vi "Periodic Tasks.vi"(8 "error in":errorcluster) -> ()   [LabVIEW 2013]
doc: "This VI runs in parallel to other tasks. It can contain as many user-defined periodic loops as you need. These can carry out PID or other sorts of timed response."
uses:
  <vilib>/Rock Robotics/WPI/Ultrasonic/WPI_UltrasonicRangeUnits.ctl
  <vilib>/Rock Robotics/SystemInterfaces/Utilities/FPGA_UtilitiesLED Source.ctl
  <vilib>/Rock Robotics/SystemInterfaces/Utilities/FPGA_UtilitiesLED State.ctl
  <vilib>/Rock Robotics/WPI/Relay/WPI_RelayValue.ctl
  <vilib>/Rock Robotics/WPI/DriverStation/WPI_DriverStationRobotMode2.ctl
  <vilib>/Rock Robotics/WPI/Solenoid/WPI_SolenoidValue.ctl
  <vilib>/Rock Robotics/WPI/Compressor/WPI_CompressorGetSetRefNum.vi
  Robot Global Data.vi
  <vilib>/Rock Robotics/WPI/Solenoid/WPI_SolenoidSetEnum.vi
panel:
  out "Shooter up":bool
  in  "Winch":bool
  in  "Bola coletada?":bool
  in  "Em posicao?":bool
  in  "upper limit":dbl=100.0
  in  "lower limit":dbl=60.0
  in  "milliseconds to wait":u32=1000
  out "Motor garra 2":dbl
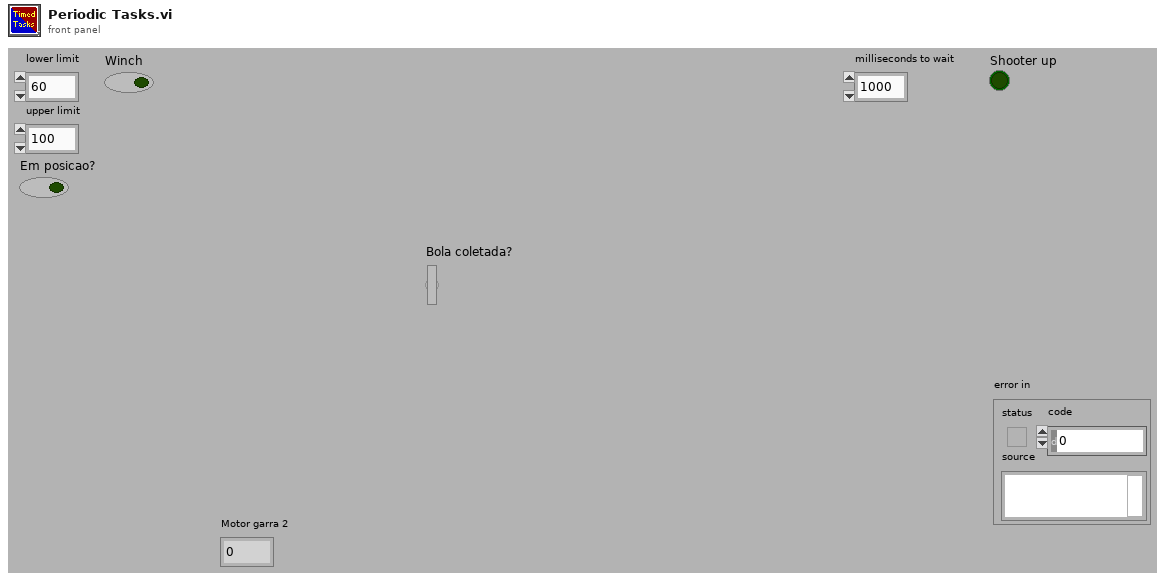
[diagram p1: front panel]
types:
  T1 = typedef "WPI_DriverStationRobotMode2.ctl" = enum16{"Autonomous Disabled", "Autonomous Enabled", "Teleop Disabled", "Teleop Enabled", "Timeout", "Finish", "Test Disabled", "Test Enabled"}
  T2 = typedef "WPI_DigitalInputDevRef.ctl" = cluster{"DevStatus":errorcluster, "DIO Channel":T3, "Digital Module":T4}
  T3 = typedef "FPGA_DIOChannel.ctl" = enum8{"DIO 1", "DIO 2", "DIO 3", "DIO 4", "DIO 5", "DIO 6", "DIO 7", "DIO 8", "DIO 9", "DIO 10", "DIO 11", "DIO 12", "DIO 13", "DIO 14", "Invalid"}
  T4 = typedef "FPGA_TypedefDigitalModule.ctl" = enum16{"Digital Module 1", "Digital Module 2"}
  T5 = typedef "WPI_MotorControlDeviceRef.ctl" = cluster{"DeviceStatus":errorcluster, "Type":enum16{"PWM", "CAN"}, "PWM":cluster{"Digital Module":T4, "PWM Channel":T6, "DeadBand":T7}, "CAN":cluster{"Device Number":u8, "Control Mode":T8, "Semaphore":T9, "Max Vout":dbl}, "Invert":bool, "TransformRef":T10, "InvTransformRef":T10}
  T6 = typedef "FPGA_DIOPWMChannel.ctl" = enum8{"PWM 1", "PWM 2", "PWM 3", "PWM 4", "PWM 5", "PWM 6", "PWM 7", "PWM 8", "PWM 9", "PWM 10", "Invalid"}
  T7 = typedef "WPI_PWMDeadband.ctl" = cluster{"Name":string, "maxPositivePwm":i32, "minPositivePwm":i32, "centerPwm":i32, "maxNegativePwm":i32, "minNegativePwm":i32, "angularRange":u16}
  T8 = typedef "WPI_CANJaguar_ControlMode.ctl" = enum8{"Percent VBus", "Current", "Speed", "Position", "Voltage"}
  T9 = typedef "Semaphore RefNum" = refnum<k1>
  T10 = typedef "WPI_PWMTransform_ConPane.ctl" = refnum<vi>
  T11 = typedef "WPI_JoystickDevRef.ctl" = cluster{"Device":T12}
  T12 = typedef "WPI_JoystickDeviceEnum.ctl" = enum16{"USB 1", "USB 2", "USB 3", "USB 4", "Kinect 1", "Kinect 2"}
  T13 = typedef "WPI_JoystickButtonState.ctl" = cluster{"Button 1":bool, "Button 2":bool, "Button 3":bool, "Button 4":bool, "Button 5":bool, "Button 6":bool, "Button 7":bool, "Button 8":bool, "Button 9":bool, "Button 10":bool, "Button 11":bool, "Button 12":bool}
  T14 = typedef "WPI_CompressorDevRef.ctl" = cluster{"DevStatus":errorcluster, "DigitalInputDevRef":T2, "RelayDevRef":T15}
  T15 = typedef "WPI_RelayDevRef.ctl" = cluster{"DevStatus":errorcluster, "Relay Channel":T16, "Digital Module":T4, "Relay Direction":T17}
  T16 = typedef "FPGA_DIORelayChannel.ctl" = enum8{"Relay 1", "Relay 2", "Relay 3", "Relay 4", "Relay 5", "Relay 6", "Relay 7", "Relay 8", "Invalid"}
  T17 = typedef "WPI_RelayDirection.ctl" = enum16{"Both directions", "Forward only", "Reverse only"}
  T18 = typedef "WPI_SolenoidValue.ctl" = enum16{"Off", "On", "Forward", "Reverse"}
  T19 = typedef "WPI_SolenoidDevRef.ctl" = cluster{"DevStatus":errorcluster, "Solenoid Module":T20, "Forward Solenoid Channel":T21, "Reverse Solenoid Channel":T21}
  T20 = typedef "FPGA_TypedefSolenoidModule.ctl" = enum16{"Solenoid Module 1", "Solenoid Module 2"}
  T21 = typedef "WPI_SolenoidChannel.ctl" = enum8{"Solenoid 1", "Solenoid 2", "Solenoid 3", "Solenoid 4", "Solenoid 5", "Solenoid 6", "Solenoid 7", "Solenoid 8", "Invalid"}
  T22 = typedef "WPI_RelayValue.ctl" = enum16{"Off", "On", "Forward", "Reverse"}
  T23 = typedef "FPGA_UtilitiesLED State.ctl" = enum16{"Off", "On", "Toggle"}
  T24 = typedef "FPGA_UtilitiesLED Source.ctl" = enum16{"User LED", "FPGA LED"}
  T25 = typedef "WPI_UltrasonicDeviceRef.ctl" = cluster{"DevStatus":errorcluster, "Ping Digital Module":T4, "Echo Digital Module":T4, "Ping Channel":T3, "Echo Channel":T3, "CntIndex":T26}
  T26 = typedef "FPGA_CounterCtrSystemIndex.ctl" = enum8{"Ctr 0", "Ctr 1", "Ctr 2", "Ctr 3", "Ctr 4", "Ctr 5", "Ctr 6", "Ctr 7", "Invalid"}
  T27 = typedef "WPI_UltrasonicRangeUnits.ctl" = enum16{"inches", "mm"}
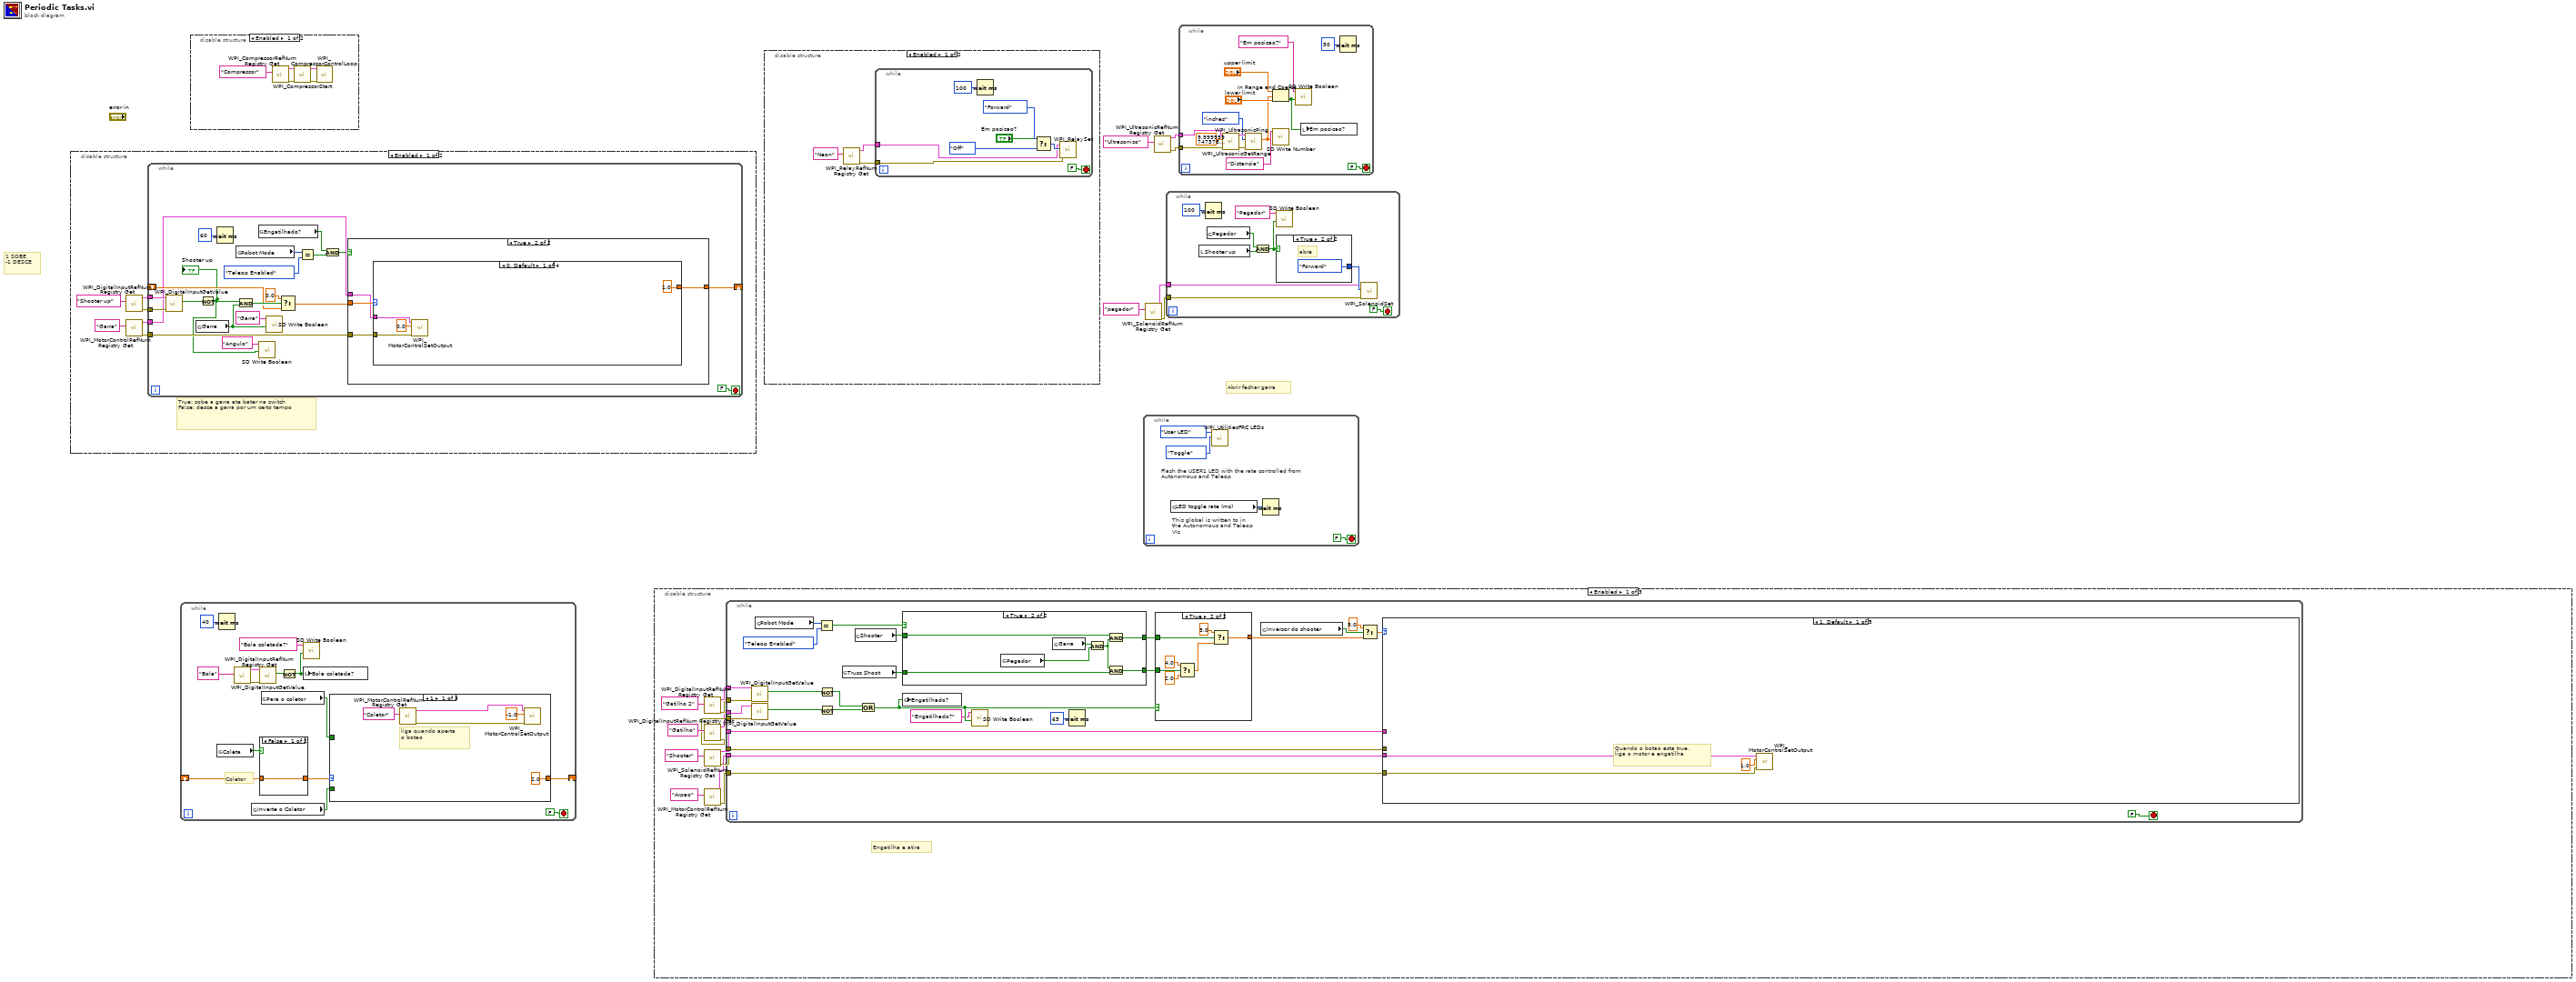
[diagram p0: block diagram]
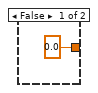
[diagram p4: hidden frame]
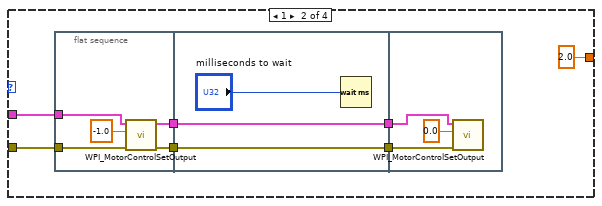
[diagram p5: hidden frame]
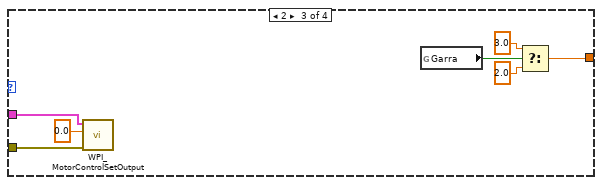
[diagram p6: hidden frame]
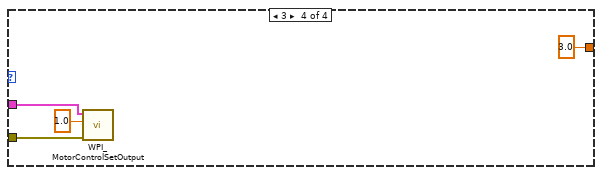
[diagram p7: hidden frame]
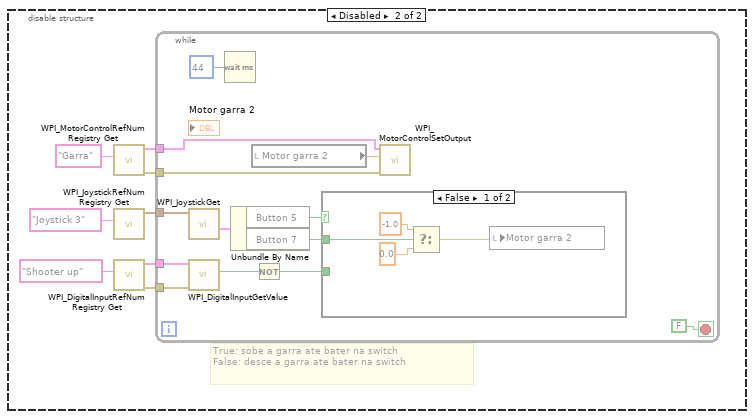
[diagram p8: hidden frame]
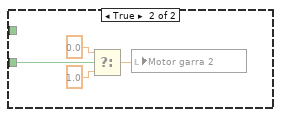
[diagram p9: hidden frame]
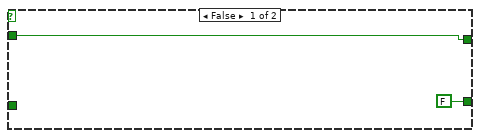
[diagram p10: hidden frame]
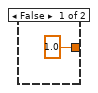
[diagram p11: hidden frame]
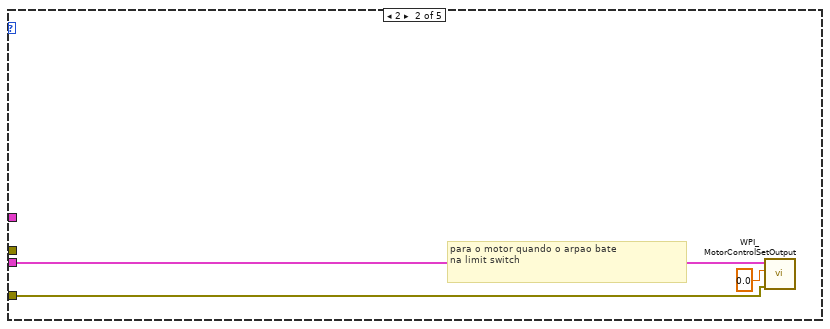
[diagram p12: hidden frame]
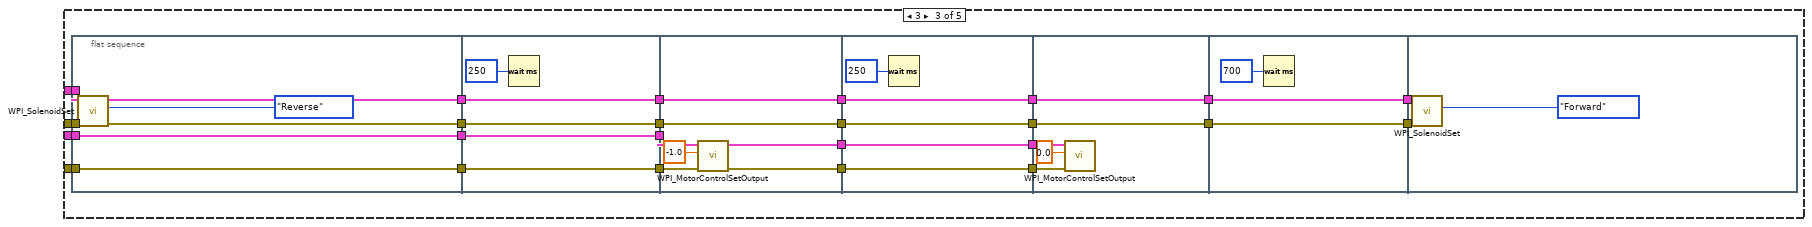
[diagram p13: hidden frame]
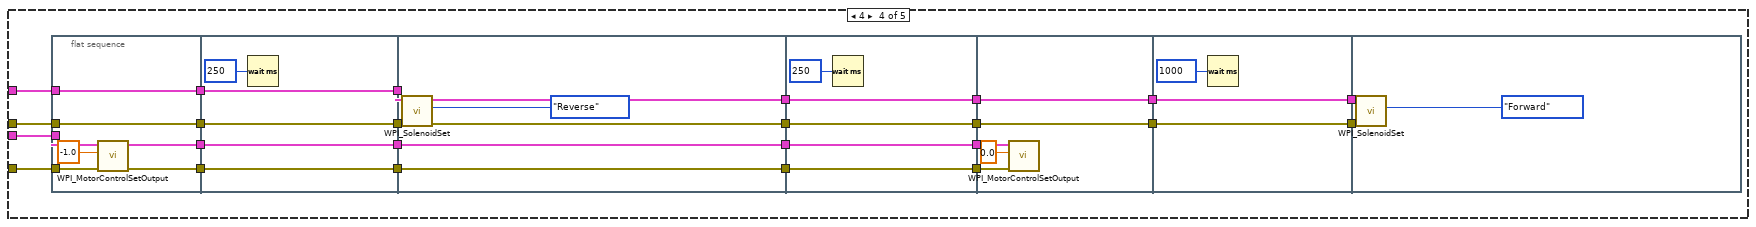
[diagram p14: hidden frame]
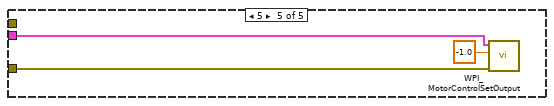
[diagram p15: hidden frame]
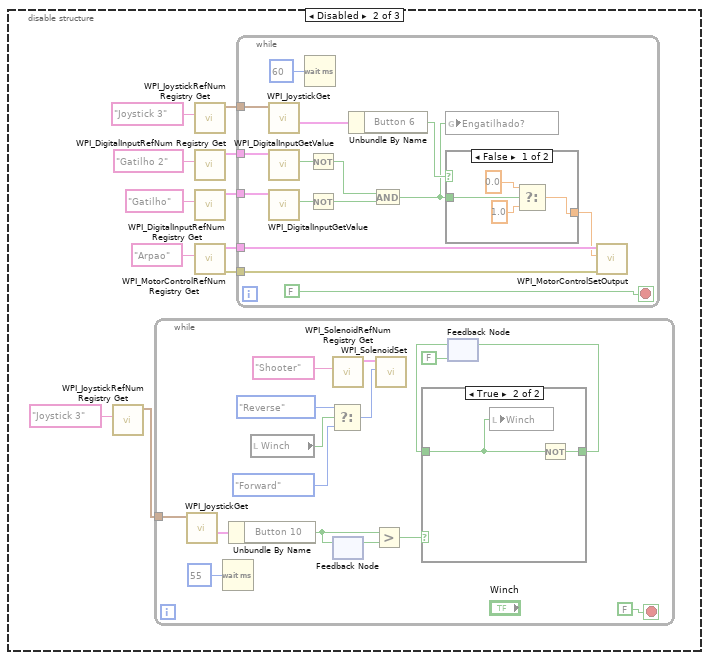
[diagram p16: hidden frame]
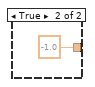
[diagram p18: hidden frame]
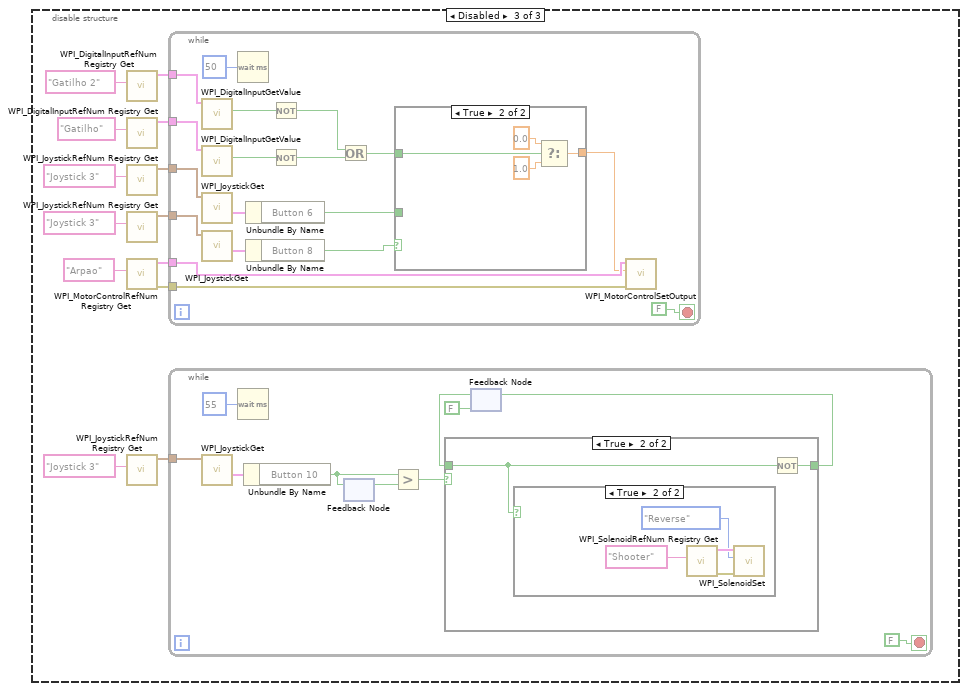
[diagram p19: hidden frame]
diagram:
  # "1 SOBE\n-1 DESCE"
  # "Abrir fechar garra"
  n1 = disable-structure shown="Enabled" {
    frame Enabled {
      # "True: sobe a garra ate bater na switch\nFalse: desce a garra por um certo tempo"
      n2 = call <vilib>:"WPI_DigitalInputRefNum Registry Get.vi"("refnum name"="Shooter up") -> ("error out"=w9:errorcluster, "DigitalInputDevRef"=w10:T2)  [unwired: 9 in]
      n3 = call <vilib>:"WPI_MotorControlRefNum Registry Get.vi"("refnum name"="Garra") -> ("error out"=w11:errorcluster, "MotorControlDevRef"=w12:T5)  [unwired: 9 in]
      n4 = while {
        tunnel: w12 -> [w24]
        tunnel: w11 -> [w23]
        tunnel: w10 -> [w32]
        tunnel: w9 -> [w31]
        shift-right: [w25] -> _
        shift-left: _ -> [w26]
        stop <- FALSE stop-if-true
        n5 = call <vilib>:"WPI_DigitalInputGetValue.vi"("error in (no error)"=w31, "DigitalInputDevRef"=w32) -> ("Value"=w22:bool)  [unwired: 7 in, 2 out]
        n6 = global read "Robot Global Data.vi" "Garra"() -> (w15:bool)
        n7 = Not(x=w22) -> (.not. x?=w13:bool)
        "Shooter up" <- w13
        n8 = Wait (ms)(milliseconds to wait=u32 60) -> ()  [unwired: 1 out]
        n9 = global read "Robot Global Data.vi" "Robot Mode"() -> (w20:T1)
        n10 = And(x=w13, y=w15) -> (x .and. y?=w29:bool)
        n11 = global read "Robot Global Data.vi" "Engatilhado?"() -> (w17:bool)
        n12 = call <vilib>:"SD Write Boolean.vi"("Boolean"=w13, "Name"="Angulo") -> ()  [unwired: 8 in, 2 out]
        n13 = call <vilib>:"SD Write Boolean.vi"("Boolean"=w15, "Name"="Garra") -> ()  [unwired: 8 in, 2 out]
        n14 = Select(t=0.0, s=w29, f=w26) -> (s? t:f=w27:dbl)
        n15 = Equal?(x=w20, y=WPI_DriverStationRobotMode2."Teleop Enabled") -> (x = y?=w18:bool)
        n16 = And(x=w17, y=w18) -> (x .and. y?=w16:bool)
        n17 = case shown="True" w16 {
          tunnel: w27 -> [_ w38]
          tunnel: [0.0 ("f") w37] -> w25
          tunnel: w24 -> [_ w36]
          tunnel: w23 -> [_ w35]
          frame False {
          }
          frame True {
            n18 = case shown="0, Default" w38 {
              tunnel: [1.0 ("Motor garra") 2.0 ("Motor garra") w65 3.0 ("f")] -> w37
              tunnel: w36 -> [w41 w48 w64 w69]
              tunnel: w35 -> [w40 w47 w63 w68]
              frame 0, Default {
                n19 = call <vilib>:"WPI_MotorControlSetOutput.vi"("error in (no error)"=w40, "Output"=0.0 ("Motor garra"), "MotorControlDevRef"=w41) -> ()  [unwired: 6 in, 3 out]
              }
              frame 1 {
                n20 = flat-sequence {
                  tunnel: w48 -> [w54]
                  tunnel: w47 -> [w53]
                  tunnel: [w51] -> w46
                  tunnel: [w50] -> w45
                  tunnel: [w57] -> w44
                  tunnel: w46 -> [w57]
                  tunnel: [w56] -> w43
                  tunnel: w45 -> [w56]
                  tunnel: w44 -> [w58]
                  tunnel: w43 -> [w60]
                  frame #0 {
                    n21 = call <vilib>:"WPI_MotorControlSetOutput.vi"("error in (no error)"=w53, "Output"=-1.0, "MotorControlDevRef"=w54) -> ("error out"=w50:errorcluster, "MotorControlDevRef"=w51:T5)  [unwired: 6 in, 1 out]
                  }
                  frame #1 {
                    n22 = Wait (ms)(milliseconds to wait="milliseconds to wait") -> ()  [unwired: 1 out]
                  }
                  frame #2 {
                    n23 = call <vilib>:"WPI_MotorControlSetOutput.vi"("error in (no error)"=w60, "Output"=0.0 ("f"), "MotorControlDevRef"=w58) -> ()  [unwired: 6 in, 3 out]
                  }
                }
              }
              frame 2 {
                n24 = call <vilib>:"WPI_MotorControlSetOutput.vi"("error in (no error)"=w63, "Output"=0.0 ("Motor garra"), "MotorControlDevRef"=w64) -> ()  [unwired: 6 in, 3 out]
                n25 = global read "Robot Global Data.vi" "Garra"() -> (w61:bool)
                n26 = Select(t=3.0, s=w61, f=2.0) -> (s? t:f=w65:dbl)
              }
              frame 3 {
                n27 = call <vilib>:"WPI_MotorControlSetOutput.vi"("error in (no error)"=w68, "Output"=1.0 ("Motor garra"), "MotorControlDevRef"=w69) -> ()  [unwired: 6 in, 3 out]
              }
            }
          }
        }
      }
    }
    frame Disabled {
      # "True: sobe a garra ate bater na switch\nFalse: desce a garra ate bater na switch"
      n28 = call <vilib>:"WPI_MotorControlRefNum Registry Get.vi"("refnum name"="Garra") -> ("error out"=w78:errorcluster, "MotorControlDevRef"=w79:T5)  [unwired: 9 in]
      n29 = call <vilib>:"WPI_JoystickRefNum Registry Get.vi"("refnum name"="Joystick 3") -> ("JoystickDevRef"=w73:T11)  [unwired: 9 in, 1 out]
      n30 = call <vilib>:"WPI_DigitalInputRefNum Registry Get.vi"("refnum name"="Shooter up") -> ("error out"=w76:errorcluster, "DigitalInputDevRef"=w77:T2)  [unwired: 9 in]
      n31 = while {
        tunnel: w79 -> [w92]
        tunnel: w78 -> [w91]
        tunnel: w77 -> [w89]
        tunnel: w76 -> [w88]
        tunnel: w73 -> [w83]
        stop <- FALSE stop-if-true
        n32 = call <vilib>:"WPI_JoystickGet.vi"("JoystickDevRef"=w83) -> ("Buttons"=w82:T13)  [unwired: 4 in, 2 out]
        n33 = call <vilib>:"WPI_DigitalInputGetValue.vi"("error in (no error)"=w88, "DigitalInputDevRef"=w89) -> ("Value"=w87:bool)  [unwired: 7 in, 2 out]
        n34 = Wait (ms)(milliseconds to wait=u32 44) -> ()  [unwired: 1 out]
        n35 = Unbundle By Name(w82) -> ("Button 5"=w81:bool, "Button 7"=w80:bool)
        n36 = local read "Motor garra 2"() -> (w85:dbl)
        n37 = Not(x=w87) -> (.not. x?=w84:bool)
        n38 = case shown="False" w81 {
          tunnel: w84 -> [_ w99]
          tunnel: w80 -> [w96 _]
          frame False {
            n39 = Select(t=-1.0, s=w96, f=0.0) -> (s? t:f=w95:dbl)
            n40 = local write "Motor garra 2"(w95) -> ()
          }
          frame True {
            n41 = Select(t=0.0, s=w99, f=1.0) -> (s? t:f=w100:dbl)
            n42 = local write "Motor garra 2"(w100) -> ()
          }
        }
        n43 = call <vilib>:"WPI_MotorControlSetOutput.vi"("error in (no error)"=w91, "Output"=w85, "MotorControlDevRef"=w92) -> ()  [unwired: 6 in, 3 out]
      }
    }
  }
  n44 = while {
    shift-right: [w113] -> _
    shift-left: _ -> [w114]
    stop <- FALSE stop-if-true
    # "Coletor"
    n45 = global read "Robot Global Data.vi" "Coleta"() -> (w107:bool)
    n46 = Wait (ms)(milliseconds to wait=u32 40) -> ()  [unwired: 1 out]
    n47 = call <vilib>:"WPI_DigitalInputRefNum Registry Get.vi"("refnum name"="Bola") -> ("error out"=w105:errorcluster, "DigitalInputDevRef"=w104:T2)  [unwired: 9 in]
    n48 = global read "Robot Global Data.vi" "Inverte o Coletor"() -> (w109:bool)
    n49 = call <vilib>:"WPI_DigitalInputGetValue.vi"("error in (no error)"=w105, "DigitalInputDevRef"=w104) -> ("Value"=w102:bool)  [unwired: 7 in, 2 out]
    n50 = case shown="False" w107 {
      tunnel: w114 -> [w115 _]
      tunnel: [w115 1.0 ("t")] -> w112
      frame False {
      }
      frame True {
      }
    }
    n51 = global read "Robot Global Data.vi" "Para o coletor"() -> (w108:bool)
    n52 = Not(x=w102) -> (.not. x?=w101:bool)
    n53 = call <vilib>:"SD Write Boolean.vi"("Boolean"=w101, "Name"="Bola coletada?") -> ()  [unwired: 8 in, 2 out]
    n54 = local write "Bola coletada?"(w101) -> ()
    n55 = case shown="1" w112 {
      selector: w112 -> [_ w127 _]
      tunnel: [2.0 ("t") w126 3.0 ("t")] -> w113
      tunnel: w108 -> [_ w124 _]
      tunnel: w109 -> [_ _ w128]
      frame 1 {
        # "liga quando aperta\no botao"
        n56 = call <vilib>:"WPI_MotorControlRefNum Registry Get.vi"("refnum name"="Coletor") -> ("error out"=w120:errorcluster, "MotorControlDevRef"=w119:T5)  [unwired: 9 in]
        n57 = call <vilib>:"WPI_MotorControlSetOutput.vi"("error in (no error)"=w120, "Output"=-1.0, "MotorControlDevRef"=w119) -> ()  [unwired: 6 in, 3 out]
      }
      frame 2 {
        # "espera o sensor \nativar"
        n58 = Or(x=w124, y="Bola coletada?") -> (x .or. y?=w123:bool)
        n59 = Select(t=3.0, s=w123, f=w127) -> (s? t:f=w126:dbl)
      }
      frame 3, Default {
        n60 = case shown="False" w128 {
          frame False {
            n61 = call <vilib>:"WPI_MotorControlRefNum Registry Get.vi"("refnum name"="Coletor") -> ("error out"=w131:errorcluster, "MotorControlDevRef"=w132:T5)  [unwired: 9 in]
            n62 = call <vilib>:"WPI_MotorControlSetOutput.vi"("error in (no error)"=w131, "Output"=0.0, "MotorControlDevRef"=w132) -> ()  [unwired: 6 in, 3 out]
          }
          frame True {
            n63 = call <vilib>:"WPI_MotorControlRefNum Registry Get.vi"("refnum name"="Coletor") -> ("error out"=w135:errorcluster, "MotorControlDevRef"=w136:T5)  [unwired: 9 in]
            n64 = call <vilib>:"WPI_MotorControlSetOutput.vi"("error in (no error)"=w135, "Output"=1.0, "MotorControlDevRef"=w136) -> ()  [unwired: 6 in, 3 out]
          }
        }
      }
    }
  }
  n65 = disable-structure shown="Enabled" {
    frame Enabled {
      n66 = call <vilib>:"WPI_CompressorRefNum Registry Get.vi"("refnum name"="Compressor") -> ("error out"=w139:errorcluster, "CompressorDevRef"=w141:T14)  [unwired: 9 in]
      n67 = call <vilib>:"WPI_CompressorStart.vi"("error in (no error)"=w139, "CompressorDevRef"=w141) -> ("error out"=w138:errorcluster, "CompressorDevRef"=w140:T14)  [unwired: 8 in]
      n68 = call <vilib>:"WPI_CompressorControlLoop.vi"("error in (no error)"=w138, "CompressorDevRef"=w140) -> ()  [unwired: 10 in]
    }
    frame Disabled {
    }
  }
  n69 = disable-structure shown="Enabled" {
    frame Enabled {
      # "Engatilha e atira"
      n70 = call <vilib>:"WPI_DigitalInputRefNum Registry Get.vi"("refnum name"="Gatilho 2") -> ("error out"=w153:errorcluster, "DigitalInputDevRef"=w154:T2)  [unwired: 9 in]
      n71 = call <vilib>:"WPI_DigitalInputRefNum Registry Get.vi"("refnum name"="Gatilho") -> ("error out"=w144:errorcluster, "DigitalInputDevRef"=w143:T2)  [unwired: 9 in]
      n72 = call <vilib>:"WPI_SolenoidRefNum Registry Get.vi"("refnum name"="Shooter") -> ("error out"=w149:errorcluster, "SolenoidDevRef"=w150:T19)  [unwired: 9 in]
      n73 = call <vilib>:"WPI_MotorControlRefNum Registry Get.vi"("refnum name"="Arpao") -> ("error out"=w147:errorcluster, "MotorControlDevRef"=w148:T5)  [unwired: 9 in]
      n74 = while {
        tunnel: w154 -> [w181]
        tunnel: w153 -> [w180]
        tunnel: w150 -> [w178]
        tunnel: w149 -> [w177]
        tunnel: w148 -> [w171]
        tunnel: w147 -> [w170]
        tunnel: w143 -> [w173]
        tunnel: w144 -> [w174]
        stop <- FALSE stop-if-true
        n75 = call <vilib>:"WPI_DigitalInputGetValue.vi"("error in (no error)"=w180, "DigitalInputDevRef"=w181) -> ("Value"=w176:bool)  [unwired: 7 in, 2 out]
        n76 = call <vilib>:"WPI_DigitalInputGetValue.vi"("error in (no error)"=w174, "DigitalInputDevRef"=w173) -> ("Value"=w167:bool)  [unwired: 7 in, 2 out]
        n77 = global read "Robot Global Data.vi" "Robot Mode"() -> (w165:T1)
        n78 = Equal?(x=w165, y=WPI_DriverStationRobotMode2."Teleop Enabled") -> (x = y?=w163:bool)
        n79 = Not(x=w176) -> (.not. x?=w172:bool)
        n80 = Not(x=w167) -> (.not. x?=w166:bool)
        n81 = global read "Robot Global Data.vi" "Truss Shoot"() -> (w160:bool)
        n82 = global read "Robot Global Data.vi" "Shooter"() -> (w162:bool)
        n83 = Or(x=w172, y=w166) -> (x .or. y?=w169:bool)
        n84 = case shown="True" w163 {
          tunnel: [w183 w190] -> w161
          tunnel: w162 -> [w183 w189]
          tunnel: w160 -> [_ w185]
          tunnel: [FALSE w187] -> w159
          frame False {
          }
          frame True {
            n85 = global read "Robot Global Data.vi" "Pegador"() -> (w184:bool)
            n86 = global read "Robot Global Data.vi" "Garra"() -> (w188:bool)
            n87 = And(x=w188, y=w184) -> (x .and. y?=w186:bool)
            n88 = And(x=w189, y=w186) -> (x .and. y?=w190:bool)
            n89 = And(x=w186, y=w185) -> (x .and. y?=w187:bool)
          }
        }
        n90 = global write "Robot Global Data.vi" "Engatilhado?"(w169) -> ()
        n91 = call <vilib>:"SD Write Boolean.vi"("Boolean"=w169, "Name"="Engatilhado?") -> ()  [unwired: 8 in, 2 out]
        n92 = Wait (ms)(milliseconds to wait=u32 65) -> ()  [unwired: 1 out]
        n93 = case shown="True" w169 {
          tunnel: [1.0 ("Output") w197] -> w157
          tunnel: w161 -> [_ w196]
          tunnel: w159 -> [_ w195]
          frame False {
          }
          frame True {
            n94 = Select(t=4.0, s=w195, f=2.0 ("Output")) -> (s? t:f=w192:dbl)
            n95 = Select(t=3.0, s=w196, f=w192) -> (s? t:f=w197:dbl)
          }
        }
        n96 = global read "Robot Global Data.vi" "Inversor do shooter"() -> (w156:bool)
        n97 = Select(t=5.0, s=w156, f=w157) -> (s? t:f=w158:dbl)
        n98 = case shown="1, Default" w158 {
          tunnel: w178 -> [_ _ w228 w270 _]
          tunnel: w177 -> [_ _ w227 w269 _]
          tunnel: w171 -> [w200 w204 w218 w272 w324]
          tunnel: w170 -> [w199 w202 w215 w271 w323]
          frame 1, Default {
            # "Quando o botao esta true, \nliga o motor e engatilha"
            n99 = call <vilib>:"WPI_MotorControlSetOutput.vi"("error in (no error)"=w199, "Output"=1.0, "MotorControlDevRef"=w200) -> ()  [unwired: 6 in, 3 out]
          }
          frame 2 {
            # "para o motor quando o arpao bate\nna limit switch"
            n100 = call <vilib>:"WPI_MotorControlSetOutput.vi"("error in (no error)"=w202, "Output"=0.0, "MotorControlDevRef"=w204) -> ()  [unwired: 6 in, 3 out]
          }
          frame 3 {
            n101 = flat-sequence {
              tunnel: [w235] -> w212
              tunnel: [w234] -> w210
              tunnel: w228 -> [w233]
              tunnel: w227 -> [w232]
              tunnel: w218 -> [w230]
              tunnel: [w230] -> w208
              tunnel: [w229] -> w206
              tunnel: w215 -> [w229]
              tunnel: w212 -> [w240]
              tunnel: [w240] -> w211
              tunnel: w210 -> [w239]
              tunnel: [w239] -> w209
              tunnel: w208 -> [w238]
              tunnel: [w238] -> w207
              tunnel: w206 -> [w237]
              tunnel: [w237] -> w205
              tunnel: w211 -> [w247]
              tunnel: [w247] -> w220
              tunnel: w209 -> [w246]
              tunnel: [w246] -> w219
              tunnel: w207 -> [w244]
              tunnel: [w243] -> w217
              tunnel: w205 -> [w242]
              tunnel: [w241] -> w213
              tunnel: w220 -> [w252]
              tunnel: [w252] -> w222
              tunnel: w219 -> [w251]
              tunnel: [w251] -> w221
              tunnel: w217 -> [w249]
              tunnel: [w249] -> w216
              tunnel: [w248] -> w214
              tunnel: w213 -> [w248]
              tunnel: [w257] -> w224
              tunnel: w222 -> [w256]
              tunnel: w221 -> [w257]
              tunnel: [w256] -> w223
              tunnel: w216 -> [w255]
              tunnel: w214 -> [w253]
              tunnel: w224 -> [w259]
              tunnel: [w259] -> w226
              tunnel: [w258] -> w225
              tunnel: w223 -> [w258]
              tunnel: w226 -> [w262]
              tunnel: w225 -> [w261]
              frame #0 {
                n102 = call-poly <vilib>:"WPI_SolenoidSet.vi"("error in (no error)"=w232, "Value"=WPI_SolenoidValue."Reverse", "SolenoidDevRef"=w233) -> ("error out"=w235:errorcluster, "SolenoidDevRef"=w234:T19)  [unwired: 7 in]
              }
              frame #1 {
                n103 = Wait (ms)(milliseconds to wait=u32 250) -> ()  [unwired: 1 out]
              }
              frame #2 {
                n104 = call <vilib>:"WPI_MotorControlSetOutput.vi"("error in (no error)"=w242, "Output"=-1.0 ("Motor shooter"), "MotorControlDevRef"=w244) -> ("error out"=w241:errorcluster, "MotorControlDevRef"=w243:T5)  [unwired: 6 in, 1 out]
              }
              frame #3 {
                n105 = Wait (ms)(milliseconds to wait=u32 250) -> ()  [unwired: 1 out]
              }
              frame #4 {
                n106 = call <vilib>:"WPI_MotorControlSetOutput.vi"("error in (no error)"=w253, "Output"=0.0 ("Motor shooter"), "MotorControlDevRef"=w255) -> ()  [unwired: 6 in, 3 out]
              }
              frame #5 {
                n107 = Wait (ms)(milliseconds to wait=u32 700) -> ()  [unwired: 1 out]
              }
              frame #6 {
                n108 = call-poly <vilib>:"WPI_SolenoidSet.vi"("error in (no error)"=w261, "Value"=WPI_SolenoidValue."Forward", "SolenoidDevRef"=w262) -> ()  [unwired: 7 in, 2 out]
              }
            }
          }
          frame 4 {
            n109 = flat-sequence {
              tunnel: [w289] -> w287
              tunnel: w270 -> [w289]
              tunnel: w269 -> [w288]
              tunnel: w272 -> [w292]
              tunnel: w271 -> [w290]
              tunnel: [w293] -> w267
              tunnel: [w291] -> w266
              tunnel: [w288] -> w265
              tunnel: [w299] -> w286
              tunnel: w287 -> [w298]
              tunnel: [w298] -> w285
              tunnel: [w297] -> w284
              tunnel: [w296] -> w283
              tunnel: w267 -> [w297]
              tunnel: w266 -> [w296]
              tunnel: w265 -> [w299]
              tunnel: w286 -> [w303]
              tunnel: [w302] -> w282
              tunnel: w285 -> [w300]
              tunnel: w284 -> [w306]
              tunnel: [w306] -> w281
              tunnel: w283 -> [w305]
              tunnel: [w305] -> w268
              tunnel: [w301] -> w264
              tunnel: w282 -> [w311]
              tunnel: [w311] -> w280
              tunnel: [w310] -> w279
              tunnel: w281 -> [w308]
              tunnel: [w308] -> w278
              tunnel: [w307] -> w277
              tunnel: w268 -> [w307]
              tunnel: w264 -> [w310]
              tunnel: [w316] -> w276
              tunnel: w280 -> [w315]
              tunnel: w279 -> [w316]
              tunnel: [w315] -> w275
              tunnel: w278 -> [w314]
              tunnel: w277 -> [w312]
              tunnel: w276 -> [w318]
              tunnel: [w318] -> w274
              tunnel: [w317] -> w273
              tunnel: w275 -> [w317]
              tunnel: w274 -> [w321]
              tunnel: w273 -> [w320]
              frame #0 {
                n110 = call <vilib>:"WPI_MotorControlSetOutput.vi"("error in (no error)"=w290, "Output"=-1.0 ("Motor shooter"), "MotorControlDevRef"=w292) -> ("error out"=w291:errorcluster, "MotorControlDevRef"=w293:T5)  [unwired: 6 in, 1 out]
              }
              frame #1 {
                n111 = Wait (ms)(milliseconds to wait=u32 250) -> ()  [unwired: 1 out]
              }
              frame #2 {
                n112 = call-poly <vilib>:"WPI_SolenoidSet.vi"("error in (no error)"=w303, "Value"=WPI_SolenoidValue."Reverse", "SolenoidDevRef"=w300) -> ("error out"=w302:errorcluster, "SolenoidDevRef"=w301:T19)  [unwired: 7 in]
              }
              frame #3 {
                n113 = Wait (ms)(milliseconds to wait=u32 250) -> ()  [unwired: 1 out]
              }
              frame #4 {
                n114 = call <vilib>:"WPI_MotorControlSetOutput.vi"("error in (no error)"=w312, "Output"=0.0 ("Motor shooter"), "MotorControlDevRef"=w314) -> ()  [unwired: 6 in, 3 out]
              }
              frame #5 {
                n115 = Wait (ms)(milliseconds to wait=u32 1000) -> ()  [unwired: 1 out]
              }
              frame #6 {
                n116 = call-poly <vilib>:"WPI_SolenoidSet.vi"("error in (no error)"=w320, "Value"=WPI_SolenoidValue."Forward", "SolenoidDevRef"=w321) -> ()  [unwired: 7 in, 2 out]
              }
            }
          }
          frame 5 {
            n117 = call <vilib>:"WPI_MotorControlSetOutput.vi"("error in (no error)"=w323, "Output"=-1.0, "MotorControlDevRef"=w324) -> ()  [unwired: 6 in, 3 out]
          }
        }
      }
    }
    frame Disabled {
      n118 = call <vilib>:"WPI_JoystickRefNum Registry Get.vi"("refnum name"="Joystick 3") -> ("JoystickDevRef"=w326:T11)  [unwired: 9 in, 1 out]
      n119 = while {
        tunnel: w326 -> [w350]
        stop <- FALSE stop-if-true
        n120 = call <vilib>:"WPI_JoystickGet.vi"("JoystickDevRef"=w350) -> ("Buttons"=w351:T13)  [unwired: 4 in, 2 out]
        n121 = Wait (ms)(milliseconds to wait=u32 55) -> ()  [unwired: 1 out]
        n122 = Unbundle By Name(w351) -> ("Button 10"=w348:bool)
        n123 = local read "Winch"() -> (w339:bool)
        n124 = Select(t=WPI_SolenoidValue."Reverse" ("Value"), s=w339, f=WPI_SolenoidValue."Forward" ("Value")) -> (s? t:f=w340:T18)
        n125 = call <vilib>:"WPI_SolenoidRefNum Registry Get.vi"("refnum name"="Shooter") -> ("SolenoidDevRef"=w342:T19)  [unwired: 9 in, 1 out]
        n126 = feedback-in #1(w348) -> ()
        n127 = feedback #1() -> (w349:bool)  [unwired: 1 in]
        n128 = Greater?(x=w348, y=w349) -> (0:w347:bool)
        n129 = call-poly <vilib>:"WPI_SolenoidSet.vi"("Value"=w340, "SolenoidDevRef"=w342) -> ()  [unwired: 8 in, 2 out]
        n130 = feedback #2(FALSE) -> (w345:bool)
        n131 = case shown="True" w347 {
          tunnel: w345 -> [w353 w354]
          tunnel: [w353 w355] -> w344
          frame False {
          }
          frame True {
            n132 = local write "Winch"(w354) -> ()
            n133 = Not(x=w354) -> (.not. x?=w355:bool)
          }
        }
        n134 = feedback-in #2(w344) -> ()
      }
      n135 = call <vilib>:"WPI_JoystickRefNum Registry Get.vi"("refnum name"="Joystick 3") -> ("JoystickDevRef"=w336:T11)  [unwired: 9 in, 1 out]
      n136 = call <vilib>:"WPI_DigitalInputRefNum Registry Get.vi"("refnum name"="Gatilho 2") -> ("DigitalInputDevRef"=w328:T2)  [unwired: 9 in, 1 out]
      n137 = call <vilib>:"WPI_DigitalInputRefNum Registry Get.vi"("refnum name"="Gatilho") -> ("DigitalInputDevRef"=w329:T2)  [unwired: 9 in, 1 out]
      n138 = call <vilib>:"WPI_MotorControlRefNum Registry Get.vi"("refnum name"="Arpao") -> ("error out"=w332:errorcluster, "MotorControlDevRef"=w333:T5)  [unwired: 9 in]
      n139 = while {
        tunnel: w336 -> [w370]
        tunnel: w333 -> [w361]
        tunnel: w332 -> [w360]
        tunnel: w329 -> [w366]
        tunnel: w328 -> [w365]
        stop <- FALSE stop-if-true
        n140 = call <vilib>:"WPI_JoystickGet.vi"("JoystickDevRef"=w370) -> ("Buttons"=w369:T13)  [unwired: 4 in, 2 out]
        n141 = call <vilib>:"WPI_DigitalInputGetValue.vi"("DigitalInputDevRef"=w365) -> ("Value"=w364:bool)  [unwired: 8 in, 2 out]
        n142 = call <vilib>:"WPI_DigitalInputGetValue.vi"("DigitalInputDevRef"=w366) -> ("Value"=w363:bool)  [unwired: 8 in, 2 out]
        n143 = Wait (ms)(milliseconds to wait=u32 60) -> ()  [unwired: 1 out]
        n144 = Not(x=w364) -> (.not. x?=w362:bool)
        n145 = Not(x=w363) -> (.not. x?=w357:bool)
        n146 = Unbundle By Name(w369) -> ("Button 6"=w367:bool)
        n147 = And(x=w362, y=w357) -> (x .and. y?=w356:bool)
        n148 = global write "Robot Global Data.vi" "Engatilhado?"(w356) -> ()
        n149 = case shown="False" w367 {
          tunnel: w356 -> [w374 _]
          tunnel: [w371 -1.0 ("f")] -> w359
          frame False {
            n150 = Select(t=0.0, s=w374, f=1.0) -> (s? t:f=w371:dbl)
          }
          frame True {
          }
        }
        n151 = call <vilib>:"WPI_MotorControlSetOutput.vi"("error in (no error)"=w360, "Output"=w359, "MotorControlDevRef"=w361) -> ()  [unwired: 6 in, 3 out]
      }
    }
    frame Disabled {
      n152 = call <vilib>:"WPI_DigitalInputRefNum Registry Get.vi"("refnum name"="Gatilho 2") -> ("DigitalInputDevRef"=w381:T2)  [unwired: 9 in, 1 out]
      n153 = call <vilib>:"WPI_DigitalInputRefNum Registry Get.vi"("refnum name"="Gatilho") -> ("DigitalInputDevRef"=w382:T2)  [unwired: 9 in, 1 out]
      n154 = call <vilib>:"WPI_JoystickRefNum Registry Get.vi"("refnum name"="Joystick 3") -> ("JoystickDevRef"=w385:T11)  [unwired: 9 in, 1 out]
      n155 = call <vilib>:"WPI_JoystickRefNum Registry Get.vi"("refnum name"="Joystick 3") -> ("JoystickDevRef"=w386:T11)  [unwired: 9 in, 1 out]
      n156 = call <vilib>:"WPI_MotorControlRefNum Registry Get.vi"("refnum name"="Arpao") -> ("error out"=w378:errorcluster, "MotorControlDevRef"=w379:T5)  [unwired: 9 in]
      n157 = call <vilib>:"WPI_JoystickRefNum Registry Get.vi"("refnum name"="Joystick 3") -> ("JoystickDevRef"=w376:T11)  [unwired: 9 in, 1 out]
      n158 = while {
        tunnel: w386 -> [w427]
        tunnel: w385 -> [w424]
        tunnel: w382 -> [w423]
        tunnel: w381 -> [w422]
        tunnel: w379 -> [w414]
        tunnel: w378 -> [w413]
        stop <- FALSE stop-if-true
        n159 = call <vilib>:"WPI_DigitalInputGetValue.vi"("DigitalInputDevRef"=w422) -> ("Value"=w420:bool)  [unwired: 8 in, 2 out]
        n160 = call <vilib>:"WPI_DigitalInputGetValue.vi"("DigitalInputDevRef"=w423) -> ("Value"=w421:bool)  [unwired: 8 in, 2 out]
        n161 = call <vilib>:"WPI_JoystickGet.vi"("JoystickDevRef"=w424) -> ("Buttons"=w425:T13)  [unwired: 4 in, 2 out]
        n162 = call <vilib>:"WPI_JoystickGet.vi"("JoystickDevRef"=w427) -> ("Buttons"=w426:T13)  [unwired: 4 in, 2 out]
        n163 = Wait (ms)(milliseconds to wait=u32 50) -> ()  [unwired: 1 out]
        n164 = Unbundle By Name(w425) -> ("Button 6"=w411:bool)
        n165 = Unbundle By Name(w426) -> ("Button 8"=w419:bool)
        n166 = Not(x=w420) -> (.not. x?=w417:bool)
        n167 = Not(x=w421) -> (.not. x?=w418:bool)
        n168 = Or(x=w417, y=w418) -> (x .or. y?=w416:bool)
        n169 = case shown="True" w419 {
          tunnel: w416 -> [_ w433]
          tunnel: [w428 w432] -> w412
          tunnel: w411 -> [w429 _]
          frame False {
            n170 = Select(t=-1.0, s=w429, f=0.0) -> (s? t:f=w428:dbl)
          }
          frame True {
            n171 = Select(t=0.0, s=w433, f=1.0) -> (s? t:f=w432:dbl)
          }
        }
        n172 = call <vilib>:"WPI_MotorControlSetOutput.vi"("error in (no error)"=w413, "Output"=w412, "MotorControlDevRef"=w414) -> ()  [unwired: 6 in, 3 out]
      }
      n173 = while {
        tunnel: w376 -> [w396]
        stop <- FALSE stop-if-true
        n174 = call <vilib>:"WPI_JoystickGet.vi"("JoystickDevRef"=w396) -> ("Buttons"=w397:T13)  [unwired: 4 in, 2 out]
        n175 = Wait (ms)(milliseconds to wait=u32 55) -> ()  [unwired: 1 out]
        n176 = Unbundle By Name(w397) -> ("Button 10"=w394:bool)
        n177 = feedback-in #3(w394) -> ()
        n178 = feedback #3() -> (w395:bool)  [unwired: 1 in]
        n179 = Greater?(x=w394, y=w395) -> (0:w393:bool)
        n180 = feedback #4(FALSE) -> (w391:bool)
        n181 = case shown="True" w393 {
          tunnel: w391 -> [w399 w400]
          tunnel: [w399 w401] -> w390
          frame False {
          }
          frame True {
            n182 = case shown="True" w400 {
              frame False {
                n183 = call <vilib>:"WPI_SolenoidRefNum Registry Get.vi"("refnum name"="Shooter") -> ("error out"=w403:errorcluster, "SolenoidDevRef"=w404:T19)  [unwired: 9 in]
                n184 = call-poly <vilib>:"WPI_SolenoidSet.vi"("error in (no error)"=w403, "Value"=WPI_SolenoidValue."Forward", "SolenoidDevRef"=w404) -> ()  [unwired: 7 in, 2 out]
              }
              frame True {
                n185 = call <vilib>:"WPI_SolenoidRefNum Registry Get.vi"("refnum name"="Shooter") -> ("error out"=w407:errorcluster, "SolenoidDevRef"=w408:T19)  [unwired: 9 in]
                n186 = call-poly <vilib>:"WPI_SolenoidSet.vi"("error in (no error)"=w407, "Value"=WPI_SolenoidValue."Reverse", "SolenoidDevRef"=w408) -> ()  [unwired: 7 in, 2 out]
              }
            }
            n187 = Not(x=w400) -> (.not. x?=w401:bool)
          }
        }
        n188 = feedback-in #4(w390) -> ()
      }
    }
  }
  n189 = disable-structure shown="Enabled" {
    frame Enabled {
      n190 = call <vilib>:"WPI_RelayRefNum Registry Get.vi"("refnum name"="Neon") -> ("error out"=w436:errorcluster, "RelayDevRef"=w437:T15)  [unwired: 9 in]
      n191 = while {
        tunnel: w437 -> [w441]
        tunnel: w436 -> [w440]
        stop <- FALSE stop-if-true
        n192 = Wait (ms)(milliseconds to wait=u32 100) -> ()  [unwired: 1 out]
        n193 = Select(t=WPI_RelayValue."Forward" ("RelayValue"), s="Em posicao?", f=WPI_RelayValue."Off" ("RelayValue")) -> (s? t:f=w443:T22)
        n194 = call <vilib>:"WPI_RelaySet.vi"("error in (no error)"=w440, "RelayValue"=w443, "RelayDevRef"=w441) -> ()  [unwired: 7 in, 2 out]
      }
    }
    frame Disabled {
    }
  }
  n195 = while {
    stop <- FALSE stop-if-true
    # "This global is written to in the Autonomous and Teleop VIs"
    # "Flash the USER1 LED with the rate controlled from Autonomous and Teleop"
    n196 = global read "Robot Global Data.vi" "LED toggle rate (ms)"() -> (w447:u32)
    n197 = call <vilib>:"WPI_UtilitiesFRC LEDs.vi"("State"=FPGA_UtilitiesLED_State."Toggle", "LED Type"=FPGA_UtilitiesLED_Source."User LED") -> ()  [unwired: 1 in, 9 out]
    n198 = Wait (ms)(milliseconds to wait=w447) -> ()  [unwired: 1 out]
  }
  n199 = call <vilib>:"WPI_SolenoidRefNum Registry Get.vi"("refnum name"="pegador") -> ("error out"=w5:errorcluster, "SolenoidDevRef"=w6:T19)  [unwired: 9 in]
  n200 = call <vilib>:"WPI_UltrasonicRefNum Registry Get.vi"("refnum name"="Ultrasonico") -> ("error out"=w2:errorcluster, "UltrasonicDevRef"=w1:T25)  [unwired: 9 in]
  n201 = while {
    tunnel: w6 -> [w457]
    tunnel: w5 -> [w456]
    stop <- FALSE stop-if-true
    n202 = local read "Shooter up"() -> (w451:bool)
    n203 = Wait (ms)(milliseconds to wait=u32 100) -> ()  [unwired: 1 out]
    n204 = global read "Robot Global Data.vi" "Pegador"() -> (w452:bool)
    n205 = And(x=w452, y=w451) -> (x .and. y?=w453:bool)
    n206 = call <vilib>:"SD Write Boolean.vi"("Boolean"=w453, "Name"="Pegador") -> ()  [unwired: 8 in, 2 out]
    n207 = case shown="True" w453 {
      tunnel: [WPI_SolenoidValue."Reverse" ("Value") WPI_SolenoidValue."Forward" ("Value")] -> w458
      frame False {
        # "fecha"
      }
      frame True {
        # "abre"
      }
    }
    n208 = call-poly <vilib>:"WPI_SolenoidSet.vi"("error in (no error)"=w456, "Value"=w458, "SolenoidDevRef"=w457) -> ()  [unwired: 7 in, 2 out]
  }
  n209 = while {
    tunnel: w1 -> [w471]
    tunnel: w2 -> [w470]
    stop <- FALSE stop-if-true
    n210 = call <vilib>:"WPI_UltrasonicPing.vi"("error in (no error)"=w470, "pingtime (Sec)"=sgl 1e-05, "UltrasonicDevRef"=w471) -> ("error out"=w469:errorcluster, "UltrasonicDevRef"=w474:T25)  [unwired: 7 out]
    n211 = call <vilib>:"WPI_UltrasonicGetRange.vi"("error in (no error)"=w469, "Range Units"=WPI_UltrasonicRangeUnits."inches", "UltrasonicDevRef"=w474) -> ("Distance"=w463:dbl)  [unwired: 8 out]
    n212 = In Range and Coerce(upper limit="upper limit", x=w463, lower limit="lower limit") -> (In Range?=w462:bool)  [unwired: 1 out]
    n213 = call <vilib>:"SD Write Number.vi"("Numeric"=w463, "Name"="Distancia") -> ()  [unwired: 8 in, 2 out]
    n214 = call <vilib>:"SD Write Boolean.vi"("Boolean"=w462, "Name"="Em posicao?") -> ()  [unwired: 8 in, 2 out]
    n215 = local write "Em posicao?"(w462) -> ()
    n216 = Wait (ms)(milliseconds to wait=u32 50) -> ()  [unwired: 1 out]
  }
